vi "Clock Map to Clock Array.vi"(8 "error in (no error)":errorcluster, 11 "Clock History Map in":T1) -> (0 "error out":errorcluster, 2 "Clock Conversion Array":T4[](array[typedef]), 3 "Clock History Map out":T1)   [LabVIEW 2021, in "Time_CIF_U.lvlib"]
uses:
  Time_CIF_U.lvlib
  Typedef/Clock History Map.ctl
  Typedef/Clock History.ctl
  Typedef/Timestamp Pair.ctl
  Typedef/Clock Conversion.ctl
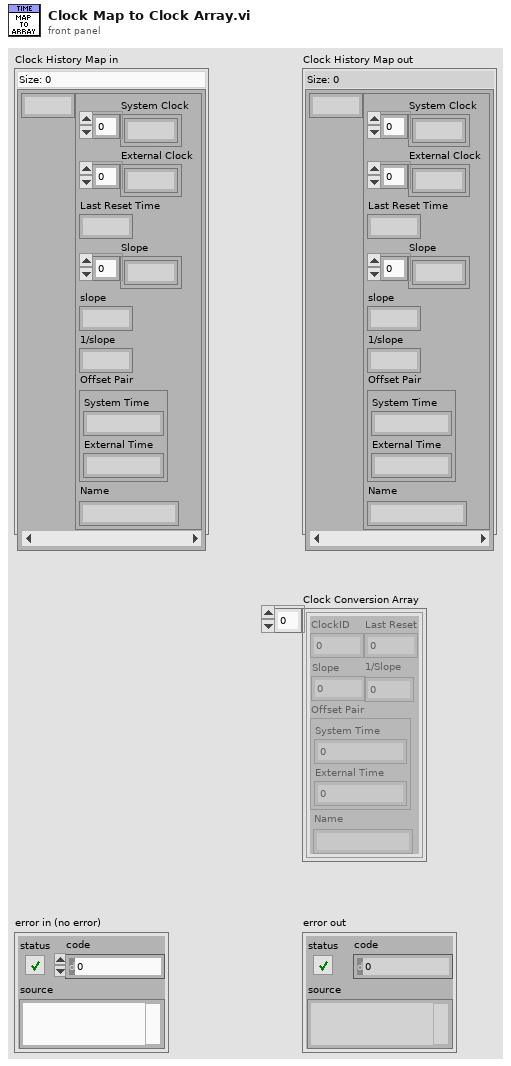
[diagram p1: front panel]
types:
  T1 = typedef "Time_CIF_U.lvlib/Clock History Map.ctl" = map{u8, T2}
  T2 = typedef "Time_CIF_U.lvlib/Clock History.ctl" = cluster{"System Clock":i64[], "External Clock":i64[], "Last Reset Time":i64, "Slope":dbl[], "slope":dbl, "1/slope":dbl, "Offset Pair":T3, "Name":string}
  T3 = typedef "Time_CIF_U.lvlib/Timestamp Pair.ctl" = cluster{"System Time":i64, "External Time":i64}
  T4 = typedef "Time_CIF_U.lvlib/Clock Conversion.ctl" = cluster{"ClockID":u8, "Last Reset":i64, "Offset Pair":T3, "Slope":dbl, "1/Slope":dbl, "Name":string}
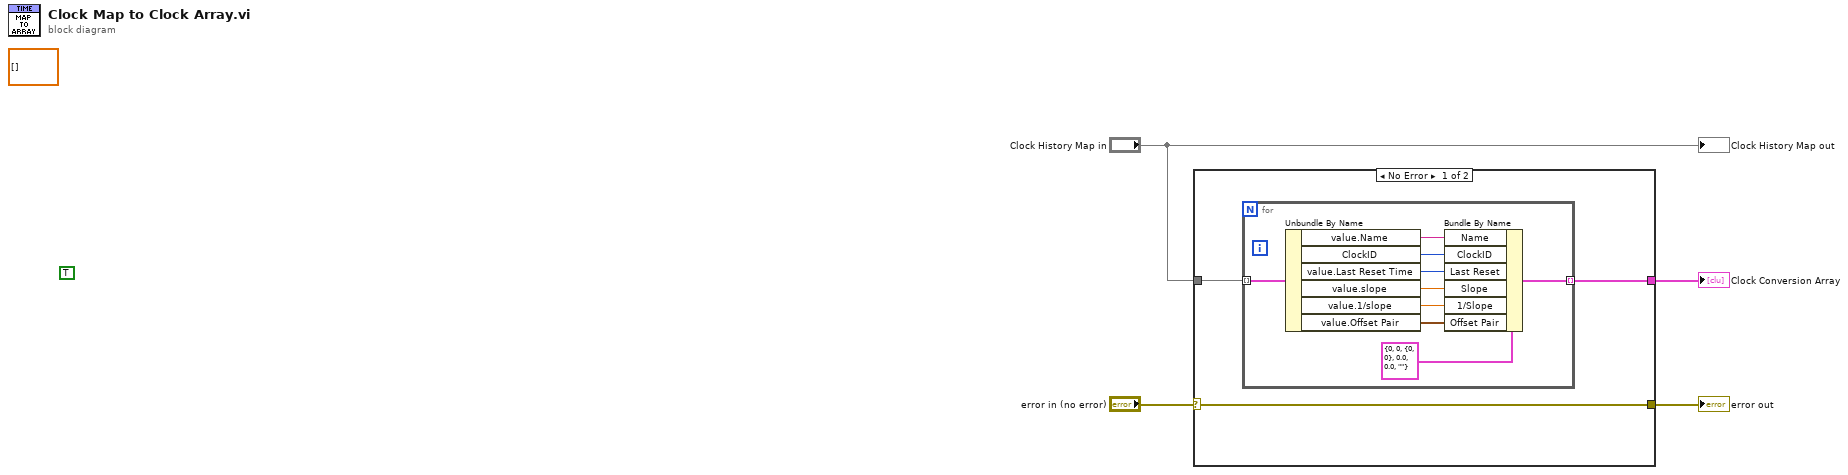
[diagram p0: block diagram]
diagram:
  (unwired) TRUE
  (unwired) dbl[][] []
  n1 = case shown="No Error" "error in (no error)" {
    selector: "error in (no error)" -> [w5 w17]
    tunnel: "Clock History Map in" -> [w7 _]
    tunnel: [w6 _] -> w3
    tunnel: [w5 w17] -> w1
    frame No Error {
      n2 = for {
        tunnel: w7 -> [w16] mode=indexing
        tunnel: [w10] -> w6 mode=indexing
        n3 = Unbundle By Name(w16) -> ("value.Name"=w9:string, "ClockID"=w14:u8, "value.Last Reset Time"=w13:i64, "value.slope"=w11:dbl, "value.1/slope"=w12:dbl, "value.Offset Pair"=w8:T3)
        n4 = Bundle By Name(cluster=T4 {"ClockID"=0, "Last Reset"=0, "Offset Pair"={"System Time"=0, "External Time"=0}, "Slope"=0.0, "1/Slope"=0.0, "Name"=""} ("Clock Conversion"), "Name"=w9, "ClockID"=w14, "Last Reset"=w13, "Slope"=w11, "1/Slope"=w12, "Offset Pair"=w8) -> (w10:T4)
      }
    }
    frame Error {
    }
  }
  "error out" <- w1
  "Clock Conversion Array" <- w3
  "Clock History Map out" <- "Clock History Map in"
